vi "Add All Calculated Channels.vi"(8 "error in (no error)":errorcluster, 9 "Calculated Channels Settings":T1, 10 "Calculated Channels":string, 11 "System Definition Ref":T8) -> (0 "error out":errorcluster, 3 ".NET Refnum out":T8)   [LabVIEW 2019, in "Simple SysDef API.lvlib"]
uses:
  <userlib>/SimpleSysDef/Simple SysDef API.lvlib
  <userlib>/SimpleSysDef/_SubVIs/System Definition Reference.ctl
  NationalInstruments.VeriStand.SystemDefinitionAPI
  <userlib>/SimpleSysDef/_SubVIs/Calculated Channels Cluster.ctl
  <userlib>/SimpleSysDef/_SubVIs/Add Calculate Channel_Formula_Settings.ctl
  <userlib>/SimpleSysDef/_SubVIs/Add Calculate Channel_Average_Settings.ctl
  <userlib>/SimpleSysDef/_SubVIs/Add Calculate Channel_Acceleration_Settings.ctl
  <userlib>/SimpleSysDef/_SubVIs/Add Calculate Channel_Maximum_Settings.ctl
  <userlib>/SimpleSysDef/_SubVIs/Add Calculate Channel_Peak and Valley_Settings.ctl
  <userlib>/SimpleSysDef/_SubVIs/Add Calculate Channel_Conditional_Settings.ctl
  <userlib>/SimpleSysDef/_SubVIs/Add Calculate Channel_Formula.vi
  <userlib>/SimpleSysDef/_SubVIs/Add Calculate Channel_Average.vi
  <userlib>/SimpleSysDef/_SubVIs/Add Calculate Channel_Acceleration.vi
  <userlib>/SimpleSysDef/_SubVIs/Add Calculate Channel_Maximum.vi
  <userlib>/SimpleSysDef/_SubVIs/Add Calculate Channel_Minimum.vi
  <userlib>/SimpleSysDef/_SubVIs/Add Calculate Channel_Peak and Valley.vi
  <userlib>/SimpleSysDef/_SubVIs/Add Calculate Channel_Conditional.vi
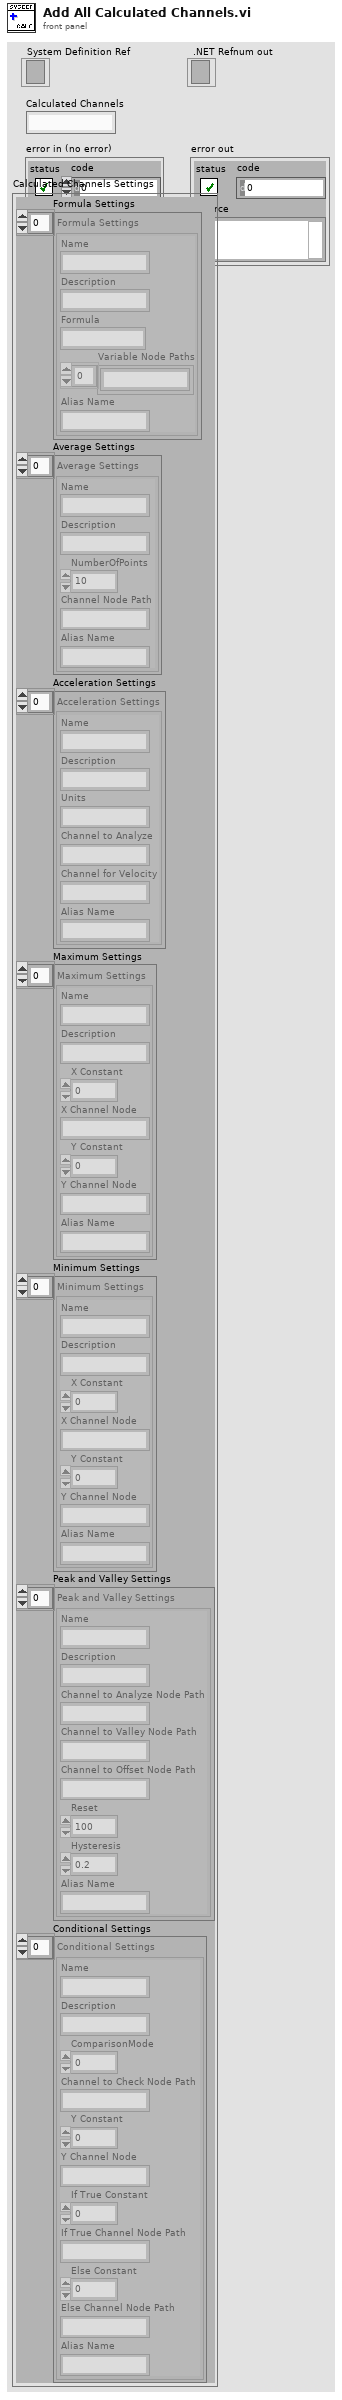
[diagram p1: front panel]
types:
  T1 = typedef "Simple SysDef API.lvlib/Calculated Channels Cluster.ctl" = cluster{"Formula Settings":T2[], "Average Settings":T3[], "Acceleration Settings":T4[], "Maximum Settings":T5[], "Minimum Settings":T5[], "Peak and Valley Settings":T6[], "Conditional Settings":T7[]}
  T2 = typedef "Simple SysDef API.lvlib/Add Calculate Channel_Formula_Settings.ctl" = cluster{"Name":string, "Description":string, "Formula":string, "Variable Node Paths":string[], "Alias Name":string}
  T3 = typedef "Simple SysDef API.lvlib/Add Calculate Channel_Average_Settings.ctl" = cluster{"Name":string, "Description":string, "NumberOfPoints":u32, "Channel Node Path":string, "Alias Name":string}
  T4 = typedef "Simple SysDef API.lvlib/Add Calculate Channel_Acceleration_Settings.ctl" = cluster{"Name":string, "Description":string, "Units":string, "Channel to Analyze":string, "Channel for Velocity":string, "Alias Name":string}
  T5 = typedef "Simple SysDef API.lvlib/Add Calculate Channel_Maximum_Settings.ctl" = cluster{"Name":string, "Description":string, "X Constant":dbl, "X Channel Node":string, "Y Constant":dbl, "Y Channel Node":string, "Alias Name":string}
  T6 = typedef "Simple SysDef API.lvlib/Add Calculate Channel_Peak and Valley_Settings.ctl" = cluster{"Name":string, "Description":string, "Channel to Analyze Node Path":string, "Channel to Valley Node Path":string, "Channel to Offset Node Path":string, "Reset":u32, "Hysteresis":dbl, "Alias Name":string}
  T7 = typedef "Simple SysDef API.lvlib/Add Calculate Channel_Conditional_Settings.ctl" = cluster{"Name":string, "Description":string, "ComparisonMode":u16, "Channel to Check Node Path":string, "Y Constant":dbl, "Y Channel Node":string, "If True Constant":dbl, "If True Channel Node Path":string, "Else Constant ":dbl, "Else Channel Node Path":string, "Alias Name":string}
  T8 = typedef "Simple SysDef API.lvlib/System Definition Reference.ctl" = refnum<k24>
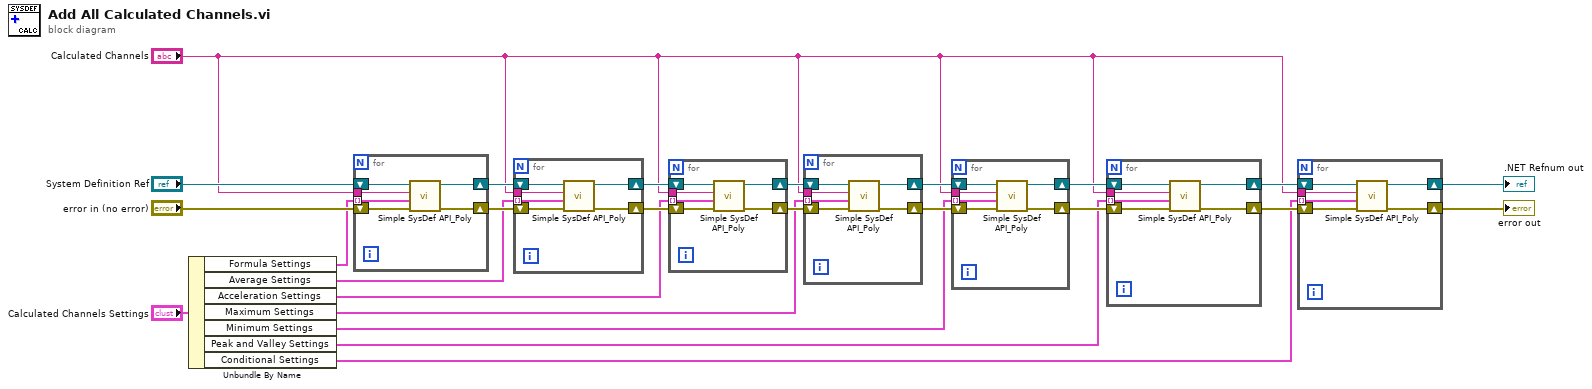
[diagram p0: block diagram]
diagram:
  n1 = Unbundle By Name("Calculated Channels Settings") -> ("Formula Settings"=w7:T2[], "Average Settings"=w6:T3[], "Acceleration Settings"=w5:T4[], "Maximum Settings"=w4:T5[], "Minimum Settings"=w3:T5[], "Peak and Valley Settings"=w2:T6[], "Conditional Settings"=w1:T7[])
  n2 = for {
    tunnel: "Calculated Channels" -> [w27]
    shift-right: [w29] -> w12
    shift-left: "error in (no error)" -> [w30]
    shift-right: [w28] -> w13
    shift-left: "System Definition Ref" -> [w31]
    tunnel: w7 -> [w26] mode=indexing
    n3 = call-poly <userlib>:"Simple SysDef API_Poly.vi"("error in (no error)"=w30, "Formula Settings"=w26, "Base Node Path"=w27, "SysDef Ref"=w31) -> ("error out"=w29:errorcluster, "SysDef Ref Out"=w28:T8)  [unwired: 5 in, 1 out]
  }
  n4 = for {
    tunnel: "Calculated Channels" -> [w33]
    shift-right: [w35] -> w14
    shift-left: w13 -> [w36]
    shift-right: [w34] -> w15
    shift-left: w12 -> [w37]
    tunnel: w6 -> [w32] mode=indexing
    n5 = call-poly <userlib>:"Simple SysDef API_Poly.vi"("error in (no error)"=w37, "Average Settings"=w32, "Base Node Path"=w33, "SysDef Ref"=w36) -> ("error out"=w34:errorcluster, "SysDef Ref Out"=w35:T8)  [unwired: 5 in, 1 out]
  }
  n6 = for {
    tunnel: "Calculated Channels" -> [w39]
    shift-right: [w41] -> w16
    shift-left: w14 -> [w43]
    shift-right: [w40] -> w17
    shift-left: w15 -> [w42]
    tunnel: w5 -> [w38] mode=indexing
    n7 = call-poly <userlib>:"Simple SysDef API_Poly.vi"("error in (no error)"=w42, "Acceleration Settings"=w38, "Base Node Path"=w39, "SysDef Ref"=w43) -> ("error out"=w40:errorcluster, "SysDef Ref Out"=w41:T8)  [unwired: 5 in, 1 out]
  }
  n8 = for {
    tunnel: "Calculated Channels" -> [w45]
    shift-right: [w47] -> w18
    shift-left: w17 -> [w48]
    shift-right: [w46] -> w19
    shift-left: w16 -> [w49]
    tunnel: w4 -> [w44] mode=indexing
    n9 = call-poly <userlib>:"Simple SysDef API_Poly.vi"("error in (no error)"=w48, "Maximum Settings"=w44, "Base Node Path"=w45, "SysDef Ref"=w49) -> ("error out"=w47:errorcluster, "SysDef Ref Out"=w46:T8)  [unwired: 5 in, 1 out]
  }
  n10 = for {
    tunnel: "Calculated Channels" -> [w51]
    shift-right: [w52] -> w20
    shift-left: w19 -> [w53]
    shift-right: [w54] -> w21
    shift-left: w18 -> [w55]
    tunnel: w3 -> [w50] mode=indexing
    n11 = call-poly <userlib>:"Simple SysDef API_Poly.vi"("error in (no error)"=w55, "Minimum Settings"=w50, "Base Node Path"=w51, "SysDef Ref"=w53) -> ("error out"=w54:errorcluster, "SysDef Ref Out"=w52:T8)  [unwired: 5 in, 1 out]
  }
  n12 = for {
    tunnel: "Calculated Channels" -> [w57]
    shift-right: [w58] -> w22
    shift-left: w20 -> [w59]
    shift-right: [w60] -> w23
    shift-left: w21 -> [w61]
    tunnel: w2 -> [w56] mode=indexing
    n13 = call-poly <userlib>:"Simple SysDef API_Poly.vi"("error in (no error)"=w61, "Peak and Valley Settings"=w56, "Base Node Path"=w57, "SysDef Ref"=w59) -> ("error out"=w60:errorcluster, "SysDef Ref Out"=w58:T8)  [unwired: 5 in, 1 out]
  }
  n14 = for {
    tunnel: "Calculated Channels" -> [w63]
    shift-right: [w64] -> w25
    shift-left: w22 -> [w65]
    shift-right: [w66] -> w24
    shift-left: w23 -> [w67]
    tunnel: w1 -> [w62] mode=indexing
    n15 = call-poly <userlib>:"Simple SysDef API_Poly.vi"("error in (no error)"=w67, "Conditional Settings"=w62, "Base Node Path"=w63, "SysDef Ref"=w65) -> ("error out"=w66:errorcluster, "SysDef Ref Out"=w64:T8)  [unwired: 5 in, 1 out]
  }
  ".NET Refnum out" <- w25
  "error out" <- w24
